vi "Get Acquisition Progress.vi"(10 "series":i32, 11 "acc":i32) -> (1 "function return":u32, 2 "series out":i32, 3 "acc out":i32)   [LabVIEW 2018, in "Copy of Andor SDK.lvlib"]
doc: "EXPNETTYPE unsigned int WINAPI GetAcquisitionProgress(long * acc, long * series);"
uses:
  Copy of Andor SDK.lvlib
  <userlib>/Andor SDK/ATMCD32D.dll
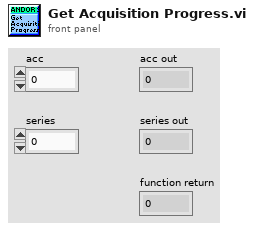
[diagram p1: front panel]
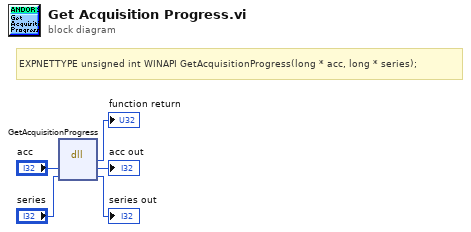
[diagram p0: block diagram]
diagram:
  # "EXPNETTYPE unsigned int WINAPI GetAcquisitionProgress(long * acc, long * series);"
  n1 = dll-call lib="C:/Program Files (x86)/National Instruments/LabVIEW 2018/user.lib/Andor SDK/ATMCD32D.*" fn="GetAcquisitionProgress"("acc"="acc", "series"="series") -> (→"function return":u32, "acc"=→"acc out":i32, "series"=→"series out":i32)  [unwired: 3 in, 2 out]
